vi "Add-action.vi"(8 "error in (no error)":errorcluster, 9 "Position in":i32, 10 "Action":refnum<class "Action.lvclass">, 11 "Sequence in":refnum<class "Action-sequence.lvclass">) -> (0 "error out":errorcluster, 1 "Position":i32, 3 "Sequence out":refnum<class "Action-sequence.lvclass">)   [LabVIEW 2013, in "PowderDeposition.lvlib" / "Action-sequence.lvclass"]
uses:
  Action-sequence.lvclass
  Action/Action.lvclass
  Action-sequence.lvclass/Action-sequence.ctl
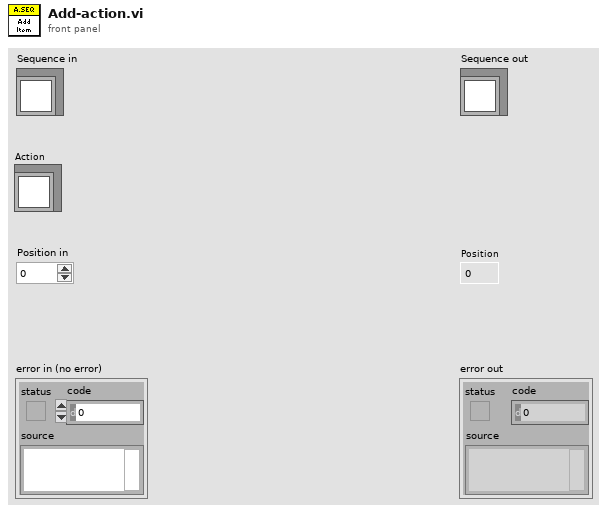
[diagram p1: front panel]
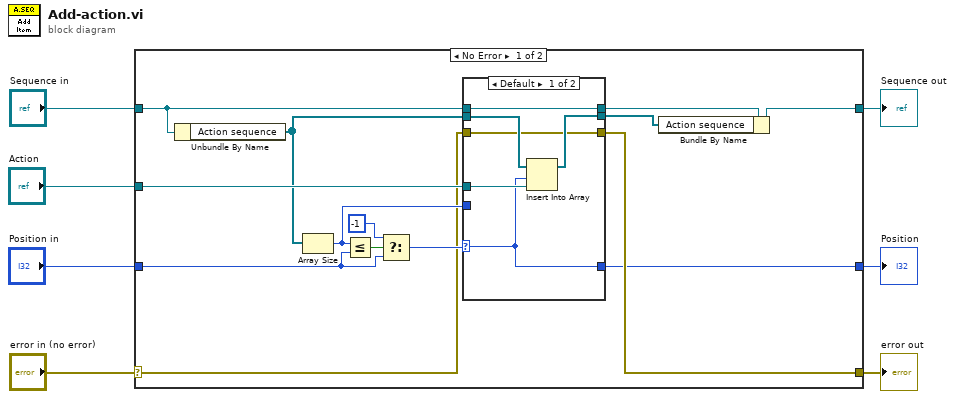
[diagram p0: block diagram]
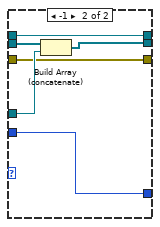
[diagram p2: hidden frame]
diagram:
  n1 = case shown="No Error" "error in (no error)" {
    selector: "error in (no error)" -> [w10 w36]
    tunnel: [w9 w36] -> w6
    tunnel: [w12 w35] -> w4
    tunnel: "Sequence in" -> [w17 w35]
    tunnel: "Action" -> [w16 _]
    tunnel: "Position in" -> [w15 w34]
    tunnel: [w8 w34] -> w1
    frame No Error {
      n2 = Unbundle By Name(w17) -> ("Action sequence"=w14:refnum<class "Action.lvclass">[])
      n3 = Array Size(array=w14) -> (size(s)=w18:i32)
      n4 = Less Or Equal?(x=w18, y=w15) -> (x <= y?=w21:bool)
      n5 = Select(t=-1, s=w21, f=w15) -> (s? t:f=w19:i32)
      n6 = case shown="Default" w19 {
        selector: w19 -> [w22 _]
        tunnel: w17 -> [w27 w30]
        tunnel: w14 -> [w26 w33]
        tunnel: w16 -> [w24 w32]
        tunnel: [w25 w31] -> w11
        tunnel: [w27 w30] -> w13
        tunnel: w10 -> [w23 w29]
        tunnel: [w23 w29] -> w9
        tunnel: w18 -> [_ w28]
        tunnel: [w22 w28] -> w8
        frame Default {
          n7 = Insert Into Array(array=w26, index=w22, new element=w24) -> (w25:refnum<class "Action.lvclass">[])
        }
        frame -1 {
          n8 = Build Array (concatenate)(w33, w32) -> (w31:refnum<class "Action.lvclass">[])
        }
      }
      n9 = Bundle By Name(cluster=w13, "Action sequence"=w11) -> (w12:refnum<class "Action-sequence.lvclass">)
    }
    frame Error {
    }
  }
  "error out" <- w6
  "Sequence out" <- w4
  "Position" <- w1
